vi "Ordenar y filtrarAlgunosPOC (SubVI).vi"(8 "Orden":bool, 9 "Columna":string="Fecha", 10 "Imeis":string[](array[string]), 11 "Tabla":string="Tabla1") -> (3 "String":string)   [LabVIEW 2012]
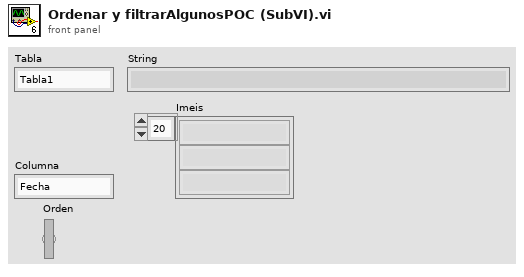
[diagram p1: front panel]
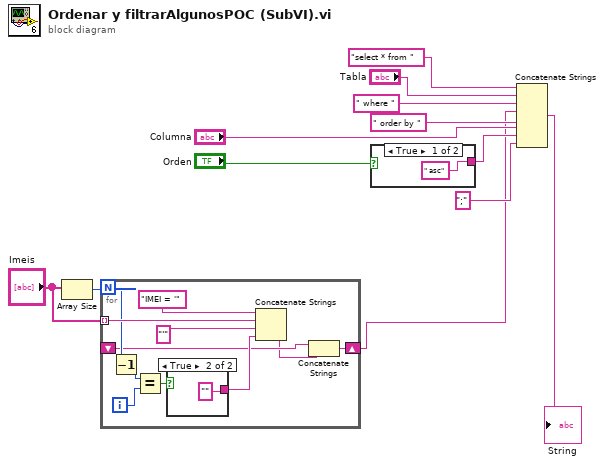
[diagram p0: block diagram]
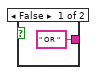
[diagram p2: hidden frame]
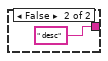
[diagram p3: hidden frame]
diagram:
  n1 = Array Size(array="Imeis") -> (size(s)=w6:i32)
  n2 = for {
    N: w6 -> [w20]
    tunnel: "Imeis" -> [w23] mode=indexing
    shift-right: [w15] -> w1
    shift-left: _ -> [w14]
    i -> [w19]
    n3 = Decrement(x=w20) -> (x-1=w18:i32)
    n4 = Equal?(x=w18, y=w19) -> (x = y?=w17:bool)
    n5 = case shown="True" w17 {
      tunnel: [" OR " ("string") "" ("string")] -> w16
      frame False {
      }
      frame True {
      }
    }
    n6 = Concatenate Strings("IMEI = '" ("string"), w23, "'" ("string"), w16) -> (w13:string)
    n7 = Concatenate Strings(w14, w13) -> (w15:string)
  }
  n8 = case shown="True" "Orden" {
    tunnel: [" asc" ("Substring") " desc" ("Substring")] -> w11
    frame True {
    }
    frame False {
    }
  }
  n9 = Concatenate Strings("select * from " ("SQL query"), "Tabla", " where " ("string"), w1, " order by " ("Substring"), "Columna", w11, ";" ("Substring")) -> (→"String":string)
